vi "Init Command.vi"(5 "Sequencer":refnum<class "MessageQ.lvclass">, 6 "Variables":refnum<class "Variables.lvclass">, 7 "VolatusAPI":refnum<class "VolatusAPI.lvclass">, 8 "error in (no error)":refnum<class "MultiErrors.lvclass">, 10 "Command Config":refnum<class "Command Config.lvclass">, 11 "Numeric Command in":refnum<class "Numeric Command.lvclass">) -> (0 "error out":refnum<class "MultiErrors.lvclass">, 3 "Numeric Command out":T1)   [LabVIEW 2020, in "VolatusSeq.lvlib" / "Numeric Command.lvclass"]
uses:
  Numeric Command.lvclass
  VolatusErrorUtilities/MultiErrors/MultiErrors.lvclass
  Command.ctl
  Volatus/MessageQ/MessageQ.lvclass
  VolatusSeqConfig/Command Type.ctl
  messages/CmdDigital/Data.ctl
  messages/CmdAnalog/Data.ctl
  Send Type.ctl
  Volatus/VolatusAPI/VolatusAPI.lvclass
  VolatusSeqConfig/Command Config/Command Config.lvclass
  VolatusSeqConfig/Numeric Command Config/Numeric Command Config.lvclass
  Volatus/VolatusAPI/VolatusAPI.lvclass/VolatusAPI.ctl
  Volatus/Module Identity/Module Identity.lvclass/Module Identity.ctl
  Volatus/Module Identity/Create.vi
  Volatus/Module Identity/Module Identity.lvclass
  C:/dev/lv20CE/relink/lv-volatus/Volatus/Identity/Identity.lvclass
  Volatus/VolatusAPI/Lookup Channel Info.vi
  <vilib>/Utility/error.llb/Error Cluster From Error Code.vi
  Volatus/VolatusAPI/Lookup Q.vi
  Numeric Command.lvclass/Numeric Command.ctl
  VolatusSeqConfig/VolatusSeqConfig.lvlib
  VolatusSeq.lvlib
  messages/CmdAnalog/CmdAnalog.lvlib
  messages/CmdDigital/CmdDigital.lvlib
  Variables/Variables.lvclass
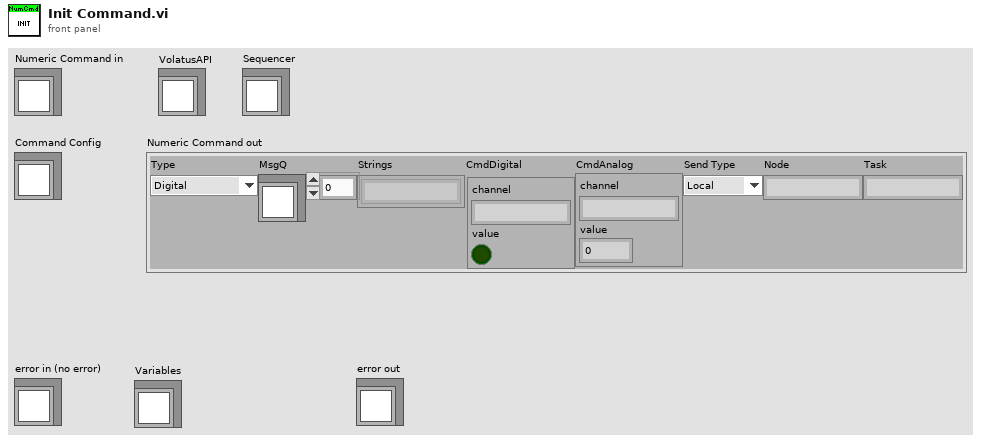
[diagram p1: front panel]
types:
  T1 = typedef "VolatusSeq.lvlib/Command.ctl" = cluster{"Type":T2, "MsgQ":refnum<class "MessageQ.lvclass">, "Strings":string[], "CmdDigital":T3, "CmdAnalog":T4, "Send Type":T5, "Node":string, "Task":string}
  T2 = typedef "VolatusSeqConfig.lvlib/Command Type.ctl" = enum16{"Digital", "Numeric", "Transition", "Stop", "StartLog", "StopLog", "Start", "Event", "Error", "HTTP"}
  T3 = typedef "CmdDigital.lvlib/Data.ctl" = cluster{"channel":string, "value":bool}
  T4 = typedef "CmdAnalog.lvlib/Data.ctl" = cluster{"channel":string, "value":dbl}
  T5 = typedef "VolatusSeq.lvlib/Send Type.ctl" = enum16{"Local", "Remote"}
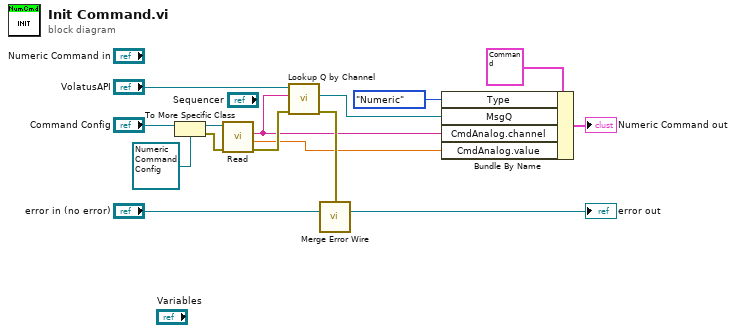
[diagram p0: block diagram]
diagram:
  n1 = To More Specific Class(target class=refnum<class "Numeric Command Config.lvclass"> refnum ("VolatusSeqConfig.lvlib:Numeric Command Config.lvclass"), reference="Command Config") -> (specific class reference=w12:refnum<class "Numeric Command Config.lvclass">, error out=w11:errorcluster)  [unwired: 1 in]
  n2 = call "Read.vi"("error in (no error)"=w11, "Numeric Command Config in"=w12) -> ("error out"=w14:errorcluster, "Command"=w2:dbl, "Channel"=w1:string)  [unwired: 6 in, 1 out]
  n3 = call "Lookup Q by Channel.vi"("error in (no error)"=w14, "Channel Name"=w1, "VolatusAPI in"="VolatusAPI") -> ("error out"=w15:errorcluster, "MessageQ"=w3:refnum<class "MessageQ.lvclass">)  [unwired: 6 in, 1 out]
  n4 = call "Merge Error Wire.vi"("error in (no error)"=w15, "MultiErrors in"="error in (no error)") -> ("MultiErrors out"=→"error out":refnum<class "MultiErrors.lvclass">)  [unwired: 13 in]
  n5 = Bundle By Name(cluster=T1 {"Type"=enum."Digital", "MsgQ"=refnum, "Strings"=[], "CmdDigital"={"channel"="", "value"=FALSE}, "CmdAnalog"={"channel"="", "value"=0.0}, "Send Type"=enum."Local", "Node"="", "Task"=""} ("Numeric Command out"), "Type"=Command_Type."Numeric", "MsgQ"=w3, "CmdAnalog.channel"=w1, "CmdAnalog.value"=w2) -> (→"Numeric Command out":T1)
